vi "Gen - Popup Single Button (Auto Close).vi"(6 "Type":enum16{"Error", "Info"}(ring)=enum."Info", 8 "Error in":errorcluster, 9 "Auto Close? F":bool, 10 "Message in":string, 11 "Header":string) -> (0 "Error out":errorcluster, 3 "OK Close":bool)   [LabVIEW 2020]
uses:
  Control/State - eFGV.ctl
panel:
  out "Type Error 2":bool
  in  "OK":bool
  out "Type Info":bool
  out "Header out":string
  in  "Exit":bool
  out "Message":string
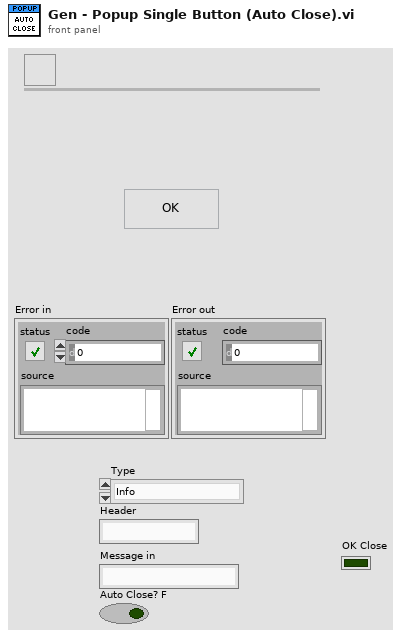
[diagram p1: front panel]
types:
  T1 = typedef "State - eFGV.ctl" = enum16{"Init", "Read", "Write", "Exit"}
  T2 = enum32{"Invalid", "Default", "Floating", "Floating/Auto-Hide", "Modal"}
  T3 = enum8{"Enabled", "Disabled", "Disabled and Grayed Out"}
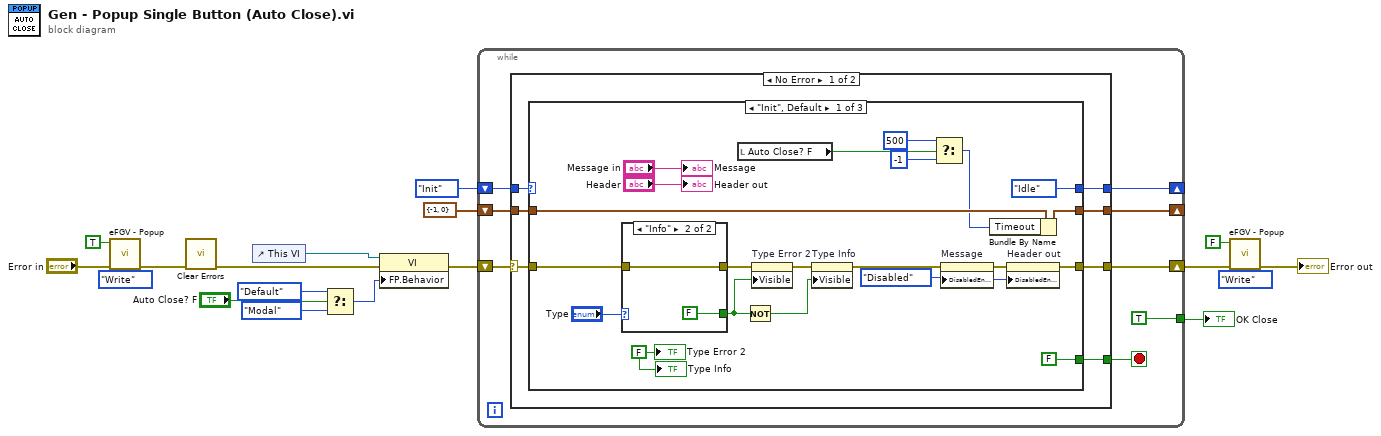
[diagram p0: block diagram]
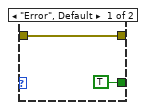
[diagram p2: hidden frame]
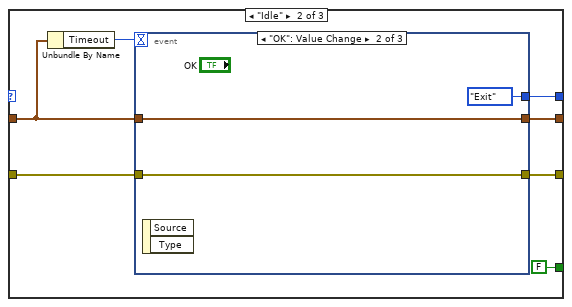
[diagram p3: hidden frame]
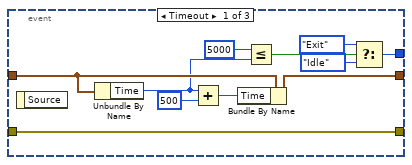
[diagram p4: hidden frame]
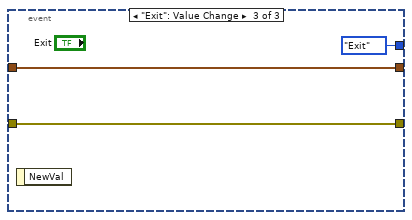
[diagram p5: hidden frame]
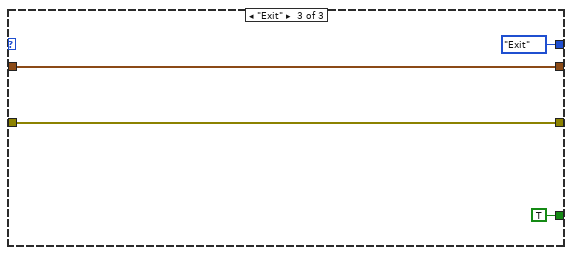
[diagram p6: hidden frame]
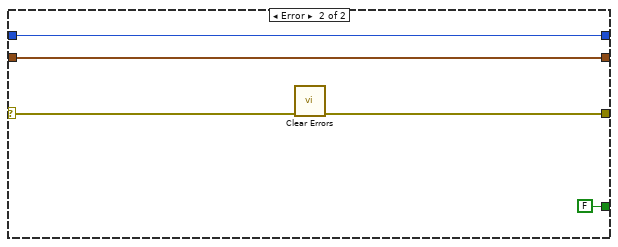
[diagram p7: hidden frame]
diagram:
  n1 = call "eFGV - Popup.vi"("Action"=State_-_eFGV."Write", "Error In"="Error in", "Popup"=TRUE) -> ("Error Out"=w5:errorcluster)  [unwired: 6 in, 2 out]
  n2 = call <vilib>:"Clear Errors.vi"("error in (no error)"=w5) -> ("error out"=w1:errorcluster)  [unwired: 5 in, 1 out]
  n3 = control-ref of="This VI"() -> (w16:refnum<vi>)
  n4 = Select(t=T2."Default" ("Front Panel Window:Behavior"), s="Auto Close? F", f=T2."Modal") -> (s? t:f=w12:T2)
  n5 = property class="VI"(reference=w16, error in=w1, "FP.Behavior"=w12) -> (error out=w15:errorcluster)  [unwired: 1 out]
  n6 = while {
    shift-right: [w24] -> _
    shift-left: enum16{"Init", "Idle", "Exit"}."Init" -> [w25]
    shift-right: [w23] -> w9
    shift-left: w15 -> [w26]
    shift-right: [w20] -> _
    shift-left: cluster{"Timeout":i32, "Time":i32} {"Timeout"=-1, "Time"=0} -> [w21]
    tunnel: [TRUE] -> w10
    stop <- w22 stop-if-true
    n7 = case shown="No Error" w26 {
      selector: w26 -> [w30 w90]
      tunnel: w25 -> [w33 w91]
      tunnel: [w32 w91] -> w24
      tunnel: [w31 w88] -> w23
      tunnel: [w29 FALSE] -> w22
      tunnel: w21 -> [w28 w87]
      tunnel: [w27 w87] -> w20
      frame No Error {
        n8 = case shown="\"Init\", Default" w33 {
          tunnel: [enum16{"Init", "Idle", "Exit"}."Idle" w65 enum16{"Init", "Idle", "Exit"}."Exit"] -> w32
          tunnel: [w39 w64 w86] -> w31
          tunnel: w30 -> [w46 w63 w86]
          tunnel: [FALSE FALSE TRUE] -> w29
          tunnel: w28 -> [w50 w60 w83]
          tunnel: [w49 w61 w83] -> w27
          frame "Init", Default {
            w42 = T3."Disabled" ("Disabled")
            w34 = FALSE ("Type Error")
            n9 = case shown="\"Info\"" "Type" {
              tunnel: [w55 w58] -> w47
              tunnel: w46 -> [w55 w58]
              tunnel: [TRUE FALSE] -> w44
              frame "Error", Default {
              }
              frame "Info" {
              }
            }
            n10 = local read "Auto Close? F"() -> (w35:bool)
            n11 = Not(x=w44) -> (.not. x?=w43:bool)
            n12 = property on="Type Error 2" class="Bool"(error in=w47, "Visible"=w44) -> (error out=w48:errorcluster)  [unwired: 1 in, 1 out]
            n13 = property on="Type Info" class="Bool (strict)"(error in=w48, "Visible"=w43) -> (error out=w40:errorcluster)  [unwired: 1 in, 1 out]
            n14 = Select(t=500 ("Timeout"), s=w35, f=-1 ("Timeout")) -> (s? t:f=w37:i32)
            n15 = property on="Message" class="Str"(error in=w40, "DisabledEnum"=w42) -> (error out=w41:errorcluster)  [unwired: 1 in, 1 out]
            n16 = Bundle By Name(cluster=w50, "Timeout"=w37) -> (w49:cluster{"Timeout":i32, "Time":i32})
            n17 = property on="Header out" class="Str"(error in=w41, "DisabledEnum"=w42) -> (error out=w39:errorcluster)  [unwired: 1 in, 1 out]
            "Message" <- "Message in"
            "Header out" <- "Header"
            "Type Info" <- w34
            "Type Error 2" <- w34
          }
          frame "Idle" {
            n18 = Unbundle By Name(w60) -> ("Timeout"=w59:i32)
            n19 = event shown="[1] \"OK\": Value Change" {
              selector: _ -> [_ _ _]
              dyn-events: _ -> [_ _ _]
              timeout: w59 -> [_ _ _]
              tunnel: [w68 enum16{"Init", "Idle", "Exit"}."Exit" enum16{"Init", "Idle", "Exit"}."Exit"] -> w65
              tunnel: [w76 w77 w80] -> w64
              tunnel: w63 -> [w76 w77 w80]
              tunnel: [w74 w78 w81] -> w61
              tunnel: w60 -> [w75 w78 w81]
              event Timeout {
                n20 = event-data() -> ()  [unwired: 1 in, 1 out]
                n21 = Unbundle By Name(w75) -> ("Time"=w71:i32)
                n22 = Add(x=w71, y=500) -> (x+y=w73:i32)
                n23 = Bundle By Name(cluster=w75, "Time"=w73) -> (w74:cluster{"Timeout":i32, "Time":i32})
                n24 = Less Or Equal?(x=5000, y=w71) -> (x <= y?=w69:bool)
                n25 = Select(t=enum16{"Init", "Idle", "Exit"}."Exit", s=w69, f=enum16{"Init", "Idle", "Exit"}."Idle") -> (s? t:f=w68:enum16{"Init", "Idle", "Exit"})
              }
              event "OK": Value Change {
                n26 = event-data() -> ()  [unwired: 1 in, 2 out]
              }
              event "Exit": Value Change {
                n27 = event-data() -> ()  [unwired: 1 in, 1 out]
              }
            }
          }
          frame "Exit" {
          }
        }
      }
      frame Error {
        n28 = call <vilib>:"Clear Errors.vi"("error in (no error)"=w90) -> ("error out"=w88:errorcluster)  [unwired: 5 in, 1 out]
      }
    }
  }
  "OK Close" <- w10
  n29 = call "eFGV - Popup.vi"("Action"=State_-_eFGV."Write", "Error In"=w9, "Popup"=FALSE) -> ("Error Out"=→"Error out":errorcluster)  [unwired: 6 in, 2 out]
